vi "ProspectivePulseTrain.vi"(4 "Counter(s)":tag="Dev1/ctr1", 5 "Source":tag="/Dev1/PFI11" caption="Trigger Source") -> (0 "error out":errorcluster, 1 "task out":refnum<k21>)   [LabVIEW 2022 SP3]
uses:
  Motion Controllers/-MotionRoutines/MotionGlobals.vi
  Pulsers/PulserGlobals.vi
  <vilib>/DAQmx/create/channels.llb/DAQmx Create Channel (CO-Pulse Generation-Frequency).vi
  <vilib>/DAQmx/configure/timing.llb/DAQmx Timing (Implicit).vi
  <vilib>/DAQmx/configure/trigger.llb/DAQmx Start Trigger (Digital Edge).vi
panel:
  in  "Trigger Edge":i32(ring)=10280 items=["Rising"=10280, "Falling"=10171]
  in  "Duty Cycle":dbl=0.1 format="%0.2f"
  # "Counter 1 output is the BNC on grey box."
  # "Trigger source comes from Aux of CTR1 (Pin 46)\n\nNeed to turn Prospective EKG modes on"
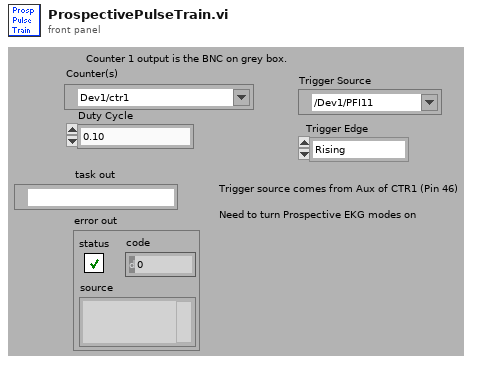
[diagram p1: front panel]
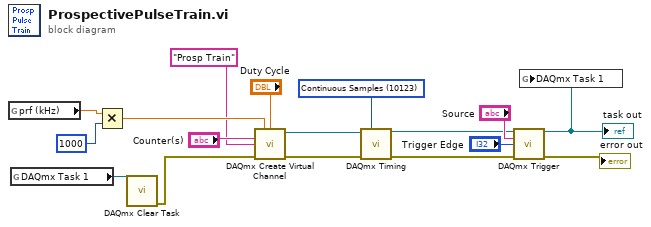
[diagram p0: block diagram]
diagram:
  w15 = 10123 items=["Finite Samples"=10178, "Continuous Samples"=10123] ("sample mode")
  n1 = global read "PulserGlobals.vi" "prf (kHz)"() -> (w1:dbl)
  n2 = global read "MotionGlobals.vi" "DAQmx Task 1"() -> (w3:refnum<k21>)
  n3 = Multiply(x=w1, y=1000) -> (x*y=w8:dbl)
  n4 = call <vilib>:"DAQmx Clear Task.vi"("task in"=w3) -> ("error out"=w4:errorcluster)  [unwired: 1 in, 13 out]
  n5 = call-poly <vilib>:"DAQmx Create Virtual Channel.vi"("frequency"=w8, "duty cycle"="Duty Cycle", "counter"="Counter(s)", "name to assign"="Prosp Train", "error in"=w4) -> ("task out"=w16:refnum<k21>, "error out"=w17:errorcluster)  [unwired: 4 in, 5 out]
  n6 = call-poly <vilib>:"DAQmx Timing.vi"("task/channels in"=w16, "sample mode"=w15, "error in"=w17) -> ("task out"=w6:refnum<k21>, "error out"=w12:errorcluster)  [unwired: 3 in, 8 out]
  n7 = call-poly <vilib>:"DAQmx Trigger.vi"("task/channels in"=w6, "source"="Source", "edge"="Trigger Edge", "error in"=w12) -> ("task out"=w5:refnum<k21>, "error out"=→"error out":errorcluster)  [unwired: 10 out]
  "task out" <- w5
  n8 = global write "MotionGlobals.vi" "DAQmx Task 1"(w5) -> ()
